vi "启动.vi"() -> ()   [LabVIEW 2016]
uses:
  <vilib>/NI/Progress Bar/Controls/Update Bar Actions.ctl
  <vilib>/NI/Progress Bar/Controls/Progress Bar Properties.ctl
  <vilib>/NI/Progress Bar/Progress Bar.lvlib
panel:
  out "exists?":bool
  out "error out":errorcluster
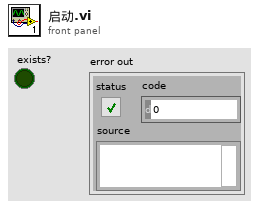
[diagram p1: front panel]
types:
  T1 = enum32{"Invalid", "Standard", "Closed", "Hidden", "Minimized", "Maximized"}
  T2 = typedef "Progress Bar.lvlib/Progress Bar Properties.ctl" = cluster{"Background Color":u32, "Installer Title":string, "Title Color":u32, "Action Text":string, "Text Color":u32, "Slider Value":u8, "Bar Color":u32, "Timeout":i32}
  T3 = typedef "Progress Bar.lvlib/Update Bar Actions.ctl" = enum16{"Add To Existing", "Set to Value"}
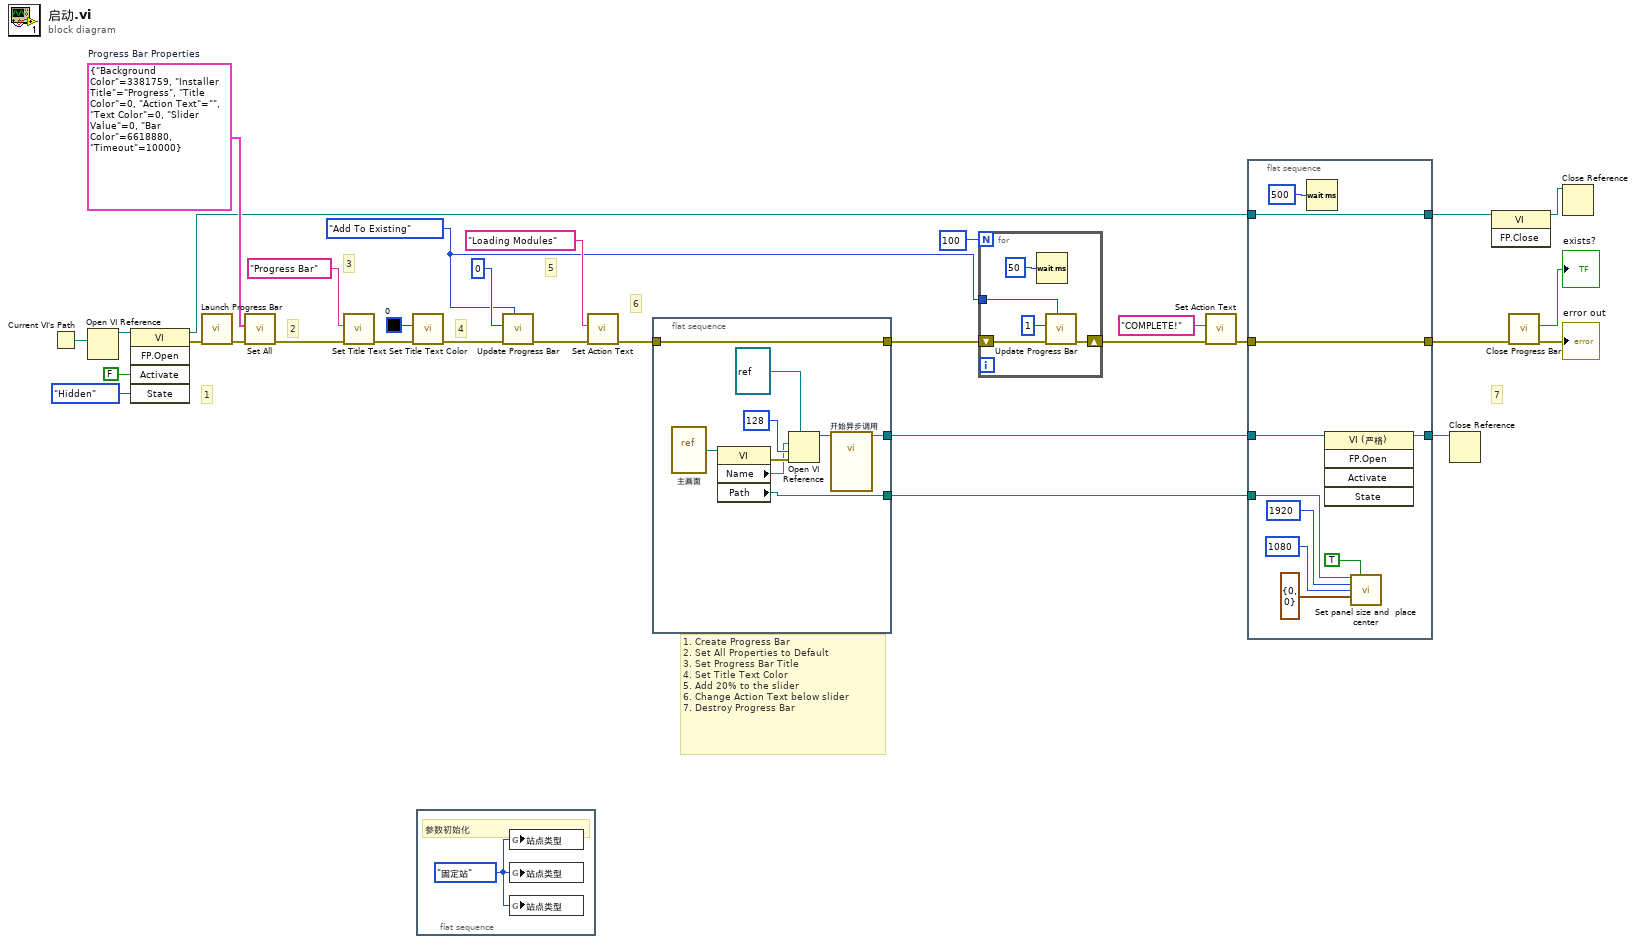
[diagram p0: block diagram]
diagram:
  w16 = T2 {"Background Color"=3381759, "Installer Title"="Progress", "Title Color"=0, "Action Text"="", "Text Color"=0, "Slider Value"=0, "Bar Color"=6618880, "Timeout"=10000}  # Progress Bar Properties
  w15 = Update_Bar_Actions."Add To Existing" ("Action")
  # "7"
  # "6"
  # "5"
  # "4"
  # "3"
  # "2"
  # "1"
  # "1. Create Progress Bar\n2. Set All Properties to Default\n3. Set Progress Bar Title\n4. Set Title Text Color\n5. Add 20% to the slider\n6. Change Action Text below slider\n7. Destroy Progress Bar"
  n1 = Current VI's Path() -> (path=w5:path)
  n2 = Open VI Reference(vi path=w5) -> (vi reference=w6:refnum<vi>)  [unwired: 5 in, 1 out]
  n3 = invoke class="VI" method="FP.Open"(reference=w6, "Activate"=FALSE ("激活？"), "State"=T1."Hidden" ("状态")) -> (reference out=w1:refnum<vi>, error out=w2:errorcluster)  [unwired: 2 in, 3 out]
  n4 = call <vilib>:"Launch Progress Bar.vi"("error in (no error)"=w2) -> ("error out"=w17:errorcluster)  [unwired: 9 in, 1 out]
  n5 = call <vilib>:"Set All.vi"("error in (no error)"=w17, "Progress Bar Properties (Default)"=w16) -> ("error out"=w27:errorcluster)  [unwired: 9 in]
  n6 = call <vilib>:"Set Title Text.vi"("error in (no error)"=w27, "Installer Title"="Progress Bar") -> ("error out"=w30:errorcluster)  [unwired: 9 in]
  n7 = call <vilib>:"Set Title Text Color.vi"("error in (no error)"=w30, "Color Box"=u32 0) -> ("error out"=w26:errorcluster)  [unwired: 9 in]
  n8 = flat-sequence {
    frame #0 {
      w32 = enum16{"微站", "固定站", "原位"}."固定站" ("站点类型")
      # "参数初始化"
      n9 = global write "VAR总磷全局变量.vi" "站点类型"(w32) -> ()
      n10 = global write "VAR总氮全局变量.vi" "站点类型"(w32) -> ()
      n11 = global write "VAR氨氮全局变量.vi" "站点类型"(w32) -> ()
    }
  }
  n12 = call <vilib>:"Update Progress Bar.vi"("Action"=w15, "error in (no error)"=w26, "Value"=u8 0) -> ("error out"=w25:errorcluster)  [unwired: 8 in]
  n13 = call <vilib>:"Set Action Text.vi"("error in (no error)"=w25, "Action Text"="Loading Modules") -> ("error out"=w24:errorcluster)  [unwired: 9 in]
  n14 = flat-sequence {
    tunnel: w24 -> [w41]
    tunnel: [w41] -> w22
    tunnel: [w40] -> w9
    tunnel: [w33] -> w7
    frame #0 {
      n15 = vi-ref "主画面.vi"() -> (w35:refnum<vi>)
      n16 = property class="VI"(reference=w35) -> (error out=w39:errorcluster, "Name"=w36:string, "Path"=w33:path)  [unwired: 1 in, 1 out]
      n17 = Open VI Reference(type specifier VI Refnum (for type only)=refnum<vi> refnum ("类型说明符VI引用句柄（仅用于类型）"), vi path=w36, options=128 ("选项"), error in (no error)=w39) -> (vi reference=w34:refnum<vi>)  [unwired: 2 in, 1 out]
      n18 = call-by-ref "开始异步调用"(reference=w34) -> (reference out=w40:refnum<vi>)  [unwired: 13 in, 1 out]
    }
  }
  n19 = for {
    N: 100 ("Value") -> [_]
    tunnel: w15 -> [w43]
    shift-right: [w46] -> w21
    shift-left: w22 -> [w45]
    n20 = Wait (ms)(milliseconds to wait=u32 50) -> ()  [unwired: 1 out]
    n21 = call <vilib>:"Update Progress Bar.vi"("Action"=w43, "error in (no error)"=w45, "Value"=u8 1) -> ("error out"=w46:errorcluster)  [unwired: 8 in]
  }
  n22 = call <vilib>:"Set Action Text.vi"("error in (no error)"=w21, "Action Text"="COMPLETE!") -> ("error out"=w20:errorcluster)  [unwired: 9 in]
  n23 = flat-sequence {
    tunnel: w20 -> [w55]
    tunnel: [w55] -> w18
    tunnel: [w54] -> w10
    tunnel: w1 -> [w54]
    tunnel: w9 -> [w53]
    tunnel: [w52] -> w8
    tunnel: w7 -> [w47]
    frame #0 {
      n24 = Wait (ms)(milliseconds to wait=u32 500) -> ()  [unwired: 1 out]
      n25 = invoke class="VI (严格)" method="FP.Open"(reference=w53) -> (reference out=w52:refnum<vi>)  [unwired: 4 in, 4 out]
      n26 = call "Set panel size and  place center.vi"("Path"=w47, "Close Reference (false)"=TRUE, "Panel Width"=1920, "Panel Height"=1080, "FP.Origin in(H & V)"=cluster{"Horizontal":i16, "Vertical":i16} {"Horizontal"=0, "Vertical"=0}) -> ()  [unwired: 6 in, 5 out]
    }
  }
  n27 = Close Reference(reference=w8) -> ()  [unwired: 1 in, 1 out]
  n28 = invoke class="VI" method="FP.Close"(reference=w10) -> (reference out=w11:refnum<vi>)  [unwired: 2 in, 2 out]
  n29 = call <vilib>:"Close Progress Bar.vi"("error in (no error)"=w18) -> ("error out"=→"error out":errorcluster, "exists?"=→"exists?":bool)  [unwired: 9 in]
  n30 = Close Reference(reference=w11) -> ()  [unwired: 1 in, 1 out]
